vi "ROIs to Mask Image.vi"(7 "Image Model":T1, 8 "Error In":errorcluster, 9 "Labels":u16[](array[numeric]), 10 "ROIs":T2[](array[typedef]) {"Contours"."Type" items=["No Selection", "Point", "Line", "Rectangle", "Oval", "Polygon", "Freehand Region", "Annulus", "Unused2", "Unused3", "Broken Line", "Freehand Line", "Rotated Rectangle"]}, 11 "Mask Image Dest":T1) -> (0 "Error Out":errorcluster, 3 "Mask Image":T1)   [LabVIEW 2021, in "Image.lvlib"]
uses:
  Image.lvlib
  <vilib>/vision/Image Controls.llb/IMAQ Image.ctl
  <vilib>/Utility/error.llb/Error Cluster From Error Code.vi
  <vilib>/ErrorRing/Error Ring.xnode
  Arrays/Arrays.lvlib
  <vilib>/vision/NI_Vision_Development_Module.lvlib
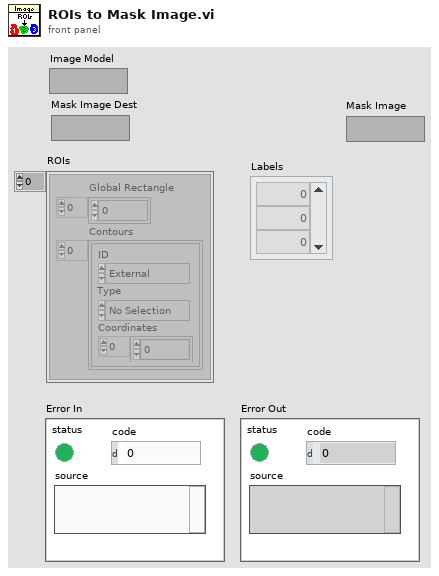
[diagram p1: front panel]
types:
  T1 = typedef "IMAQ Image.ctl" = refnum<image>
  T2 = typedef "ROI Descriptor" = cluster{"Global Rectangle":i32[], "Contours":cluster{"ID":enum32{"External", "Internal"}, "Type":u32, "Coordinates":i32[]}[]}
  T3 = typedef "Image Type" = u32
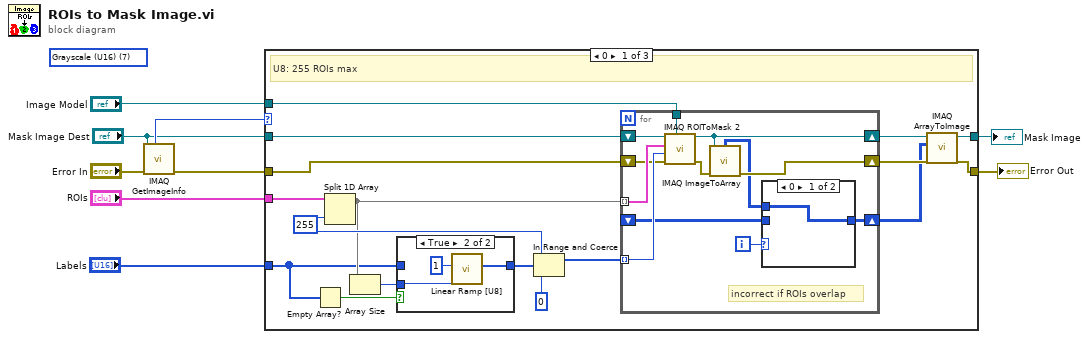
[diagram p0: block diagram]
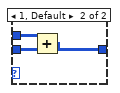
[diagram p2: hidden frame]
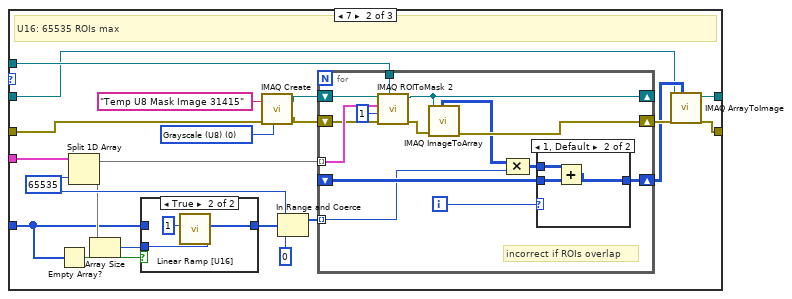
[diagram p4: hidden frame]
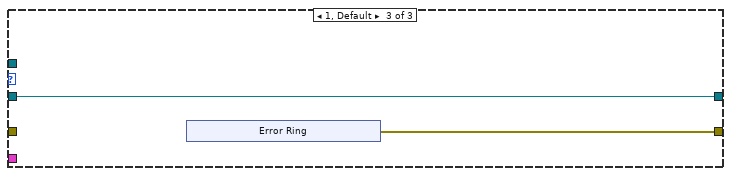
[diagram p7: hidden frame]
diagram:
  (unwired) T3 7 items=["Grayscale (U8)", "Grayscale (I16)", "Grayscale (SGL)", "Complex (CSG)", "RGB (U32)", "HSL (U32)", "RGB (U64)", "Grayscale (U16)"] ("Image Type")
  n1 = call "IMAQ GetImageInfo"("error in (no error)"="Error In", "Image"="Mask Image Dest") -> ("error out"=w6:errorcluster, "Image Type"=w8:T3)  [unwired: 2 in, 6 out]
  n2 = case shown="0" w8 {
    tunnel: "Mask Image Dest" -> [w20 w47 w90]
    tunnel: w6 -> [w16 w51 _]
    tunnel: [w11 w54 w89] -> w5
    tunnel: [w13 w56 w90] -> w4
    tunnel: "ROIs" -> [w26 w66 _]
    tunnel: "Labels" -> [w15 w57 _]
    tunnel: "Image Model" -> [w19 w60 _]
    frame 0 {
      w22 = u16 255 ("index")
      # "U8: 255 ROIs max"
      n3 = Empty Array?(array=w15) -> (empty?=w25:bool)
      n4 = Split 1D Array(array=w26, index=w22) -> (first subarray=w18:T2[])  [unwired: 1 out]
      n5 = Array Size(array=w18) -> (size(s)=w24:i32)
      n6 = case shown="True" w25 {
        tunnel: w24 -> [_ w46]
        tunnel: [w43 w45] -> w23
        tunnel: w15 -> [w43 _]
        frame False {
        }
        frame True {
          n7 = call "Linear Ramp [U8].vi"("# Elements"=w46, "Start (0)"=u8 1) -> ("Ramp"=w45:u8[])  [unwired: 7 in]
        }
      }
      n8 = In Range and Coerce(upper limit=w22, x=w23, lower limit=u16 0) -> (coerced(x)=w17:u16[])  [unwired: 1 out]
      n9 = for {
        shift-right: [w33] -> w14
        shift-left: w20 -> [w38]
        tunnel: w19 -> [w37]
        tunnel: w18 -> [w36] mode=indexing
        tunnel: w17 -> [w35] mode=indexing
        shift-right: [w28] -> w12
        shift-left: w16 -> [w34]
        shift-right: [w30] -> w10
        shift-left: _ -> [w29]
        i -> [w31]
        # "incorrect if ROIs overlap"
        n10 = call "IMAQ ROIToMask 2"("Image Model"=w37, "error in (no error)"=w34, "Filling Value (255)"=w35, "ROI Descriptor"=w36, "Image"=w38) -> ("error out"=w32:errorcluster, "Image Out"=w33:T1)  [unwired: 4 in, 1 out]
        n11 = call "IMAQ ImageToArray"("error in (no error)"=w32, "Image"=w33) -> ("error out"=w28:errorcluster, "Image Pixels (U8)"=w27:u8[][])  [unwired: 2 in, 3 out]
        n12 = case shown="0" w31 {
          tunnel: w27 -> [w39 w42]
          tunnel: [w39 w40] -> w30
          tunnel: w29 -> [_ w41]
          frame 0 {
          }
          frame 1, Default {
            n13 = Add(x=w42, y=w41) -> (x+y=w40:u8[][])
          }
        }
      }
      n14 = call "IMAQ ArrayToImage"("error in (no error)"=w12, "Image Pixels (U8)"=w10, "Image"=w14) -> ("error out"=w11:errorcluster, "Image Out"=w13:T1)  [unwired: 7 in]
    }
    frame 7 {
      w48 = T3 0 items=["Grayscale (U8)", "Grayscale (I16)", "Grayscale (SGL)", "Complex (CSG)", "RGB (U32)", "HSL (U32)", "RGB (U64)", "Grayscale (U16)"] ("Image Type")
      w62 = u16 65535 ("index")
      # "U16: 65535 ROIs max"
      n15 = Empty Array?(array=w57) -> (empty?=w65:bool)
      n16 = Split 1D Array(array=w66, index=w62) -> (first subarray=w59:T2[])  [unwired: 1 out]
      n17 = Array Size(array=w59) -> (size(s)=w64:i32)
      n18 = case shown="True" w65 {
        tunnel: w64 -> [_ w88]
        tunnel: [w85 w87] -> w63
        tunnel: w57 -> [w85 _]
        frame False {
        }
        frame True {
          n19 = call "Linear Ramp [U16].vi"("# Elements"=w88, "Start (0)"=u16 1) -> ("Ramp"=w87:u16[])  [unwired: 7 in]
        }
      }
      n20 = call "IMAQ Create"("Image Name"="Temp U8 Mask Image 31415", "Image Type"=w48, "error in (no error)"=w51) -> ("New Image"=w52:T1, "error out"=w50:errorcluster)  [unwired: 2 in]
      n21 = In Range and Coerce(upper limit=w62, x=w63, lower limit=u16 0) -> (coerced(x)=w58:u16[])  [unwired: 1 out]
      n22 = for {
        shift-right: [w76] -> _
        shift-left: w52 -> [w80]
        tunnel: w60 -> [w79]
        tunnel: w59 -> [w78] mode=indexing
        tunnel: w58 -> [w68] mode=indexing
        shift-right: [w71] -> w55
        shift-left: w50 -> [w77]
        shift-right: [w73] -> w53
        shift-left: _ -> [w72]
        i -> [w74]
        # "incorrect if ROIs overlap"
        n23 = call "IMAQ ROIToMask 2"("Image Model"=w79, "error in (no error)"=w77, "Filling Value (255)"=1, "ROI Descriptor"=w78, "Image"=w80) -> ("error out"=w75:errorcluster, "Image Out"=w76:T1)  [unwired: 4 in, 1 out]
        n24 = call "IMAQ ImageToArray"("error in (no error)"=w75, "Image"=w76) -> ("error out"=w71:errorcluster, "Image Pixels (U8)"=w67:u8[][])  [unwired: 2 in, 3 out]
        n25 = Compound Arithmetic op=MULTIPLY(w67, w68) -> (w69:u16[][])
        n26 = case shown="1, Default" w74 {
          tunnel: w69 -> [w81 w84]
          tunnel: [w81 w82] -> w73
          tunnel: w72 -> [_ w83]
          frame 0 {
          }
          frame 1, Default {
            n27 = Add(x=w84, y=w83) -> (x+y=w82:u16[][])
          }
        }
      }
      n28 = call "IMAQ ArrayToImage"("Image Pixels (U16)"=w53, "error in (no error)"=w55, "Image"=w47) -> ("error out"=w54:errorcluster, "Image Out"=w56:T1)  [unwired: 7 in]
    }
    frame 1, Default {
      n29 = xnode "Error Ring"() -> ("error out"=w89:errorcluster)
    }
  }
  "Error Out" <- w5
  "Mask Image" <- w4
